vi "CreateControlSignal.vi"(7 "V":dbl, 9 "duty cycle (%)":dbl, 11 "frequency":dbl) -> (2 "dt":dbl, 3 "Y":dbl[](array[numeric]))   [LabVIEW 2014]
uses:
  <vilib>/measure/NI_MABase.lvlib
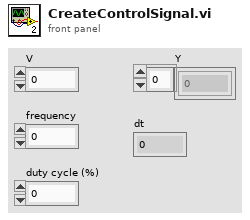
[diagram p1: front panel]
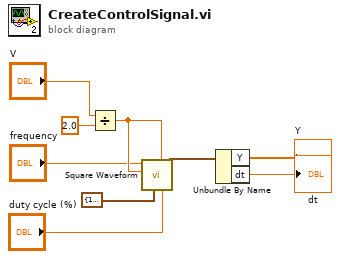
[diagram p0: block diagram]
diagram:
  n1 = Divide(x="V", y=2.0) -> (x/y=w6:dbl)
  n2 = call <vilib>:"Square Waveform.vi"("duty cycle (%)"="duty cycle (%)", "offset"=w6, "sampling info"=cluster{"Fs":dbl, "#s":dbl} {"Fs"=100000.0, "#s"=10000.0}, "amplitude"=w6, "frequency"="frequency") -> ("signal out"=w7:waveform(dbl))  [unwired: 5 in, 1 out]
  n3 = Unbundle By Name(w7) -> ("Y"=→"Y":dbl[], "dt"=→"dt":dbl)
